vi "Test Parser Compatibility.vi"(8 "error in":errorcluster) -> (0 "error out":errorcluster)   [LabVIEW 2019]
uses:
  lvsrc/Classes/Parse/ParseVectorFile/ParseVectorFile.lvclass
  C:/Program Files (x86)/National Instruments/LabVIEW 2019/vi.lib/JKI/JKI SMO/SMO/SMO.lvclass
  <vilib>/addons/_JKI Toolkits/Caraya/classes/Assert/Assert True.vi
  <vilib>/Utility/AggHandler/Cls_AggHandler.xnode
  lvsrc/subVIs/typedefs/Parsed Path - Cluster.ctl
  <vilib>/Analysis/Matrix/Datatypes/RealMatrix.ctl
  lvsrc/subVIs/typedefs/Parsed Funnel - Cluster.ctl
  lvsrc/subVIs/typedefs/Parsed Rect - Cluster.ctl
  lvsrc/Classes/Parse/Dot/Dot.lvclass
  <vilib>/JKI/JKI SMO/SMO/SMO.lvclass
  <vilib>/addons/_JKI Toolkits/Caraya/classes/Test/Test.lvclass
  <vilib>/addons/_JKI Toolkits/Caraya/classes/Assert/Assert.lvclass
  <vilib>/Analysis/Matrix/NI_Matrix.lvlib
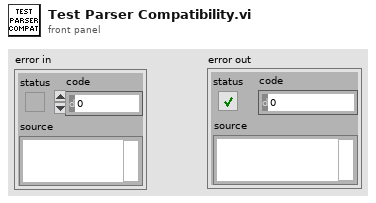
[diagram p1: front panel]
types:
  T1 = typedef "ParseVectorFile.lvclass/PublicEvents--ParseVectorFile.ParsedData.ctl" = cluster{"Paths":refnum<class "Path.lvclass">[], "Rectangles":refnum<class "Rectangle.lvclass">[], "SVGImage":refnum<class "SVGImage.lvclass">, "Dots":refnum<class "Dot.lvclass">[]}
  T2 = typedef "Parsed Path - Cluster.ctl" = cluster{"Fill Color":string, "Stroke Color":string, "Commands":cluster{"Command Type":string, "Coordinates":cluster{"X":dbl, "Y":dbl}[]}[], "Transformation Matrix":T3}
  T3 = typedef "NI_Matrix.lvlib/RealMatrix.ctl" = dbl[][]
  T4 = typedef "Parsed Funnel - Cluster.ctl" = cluster{"Fill Color":string, "Stroke Color":string, "Commands":cluster{"Command Type":string, "Coordinates":cluster{"X":dbl, "Y":dbl}[]}[], "Transformation Matrix":T3}
  T5 = typedef "Parsed Rect - Cluster.ctl" = cluster{"Fill":string, "Stroke":string, "width":dbl, "height":dbl, "x":dbl, "y":dbl, "Transformation Matrix":T3}
  T6 = cluster{" paths":T2[], " funnels":T4[], "rects":T5[], "Dots":refnum<class "Dot.lvclass">[]}
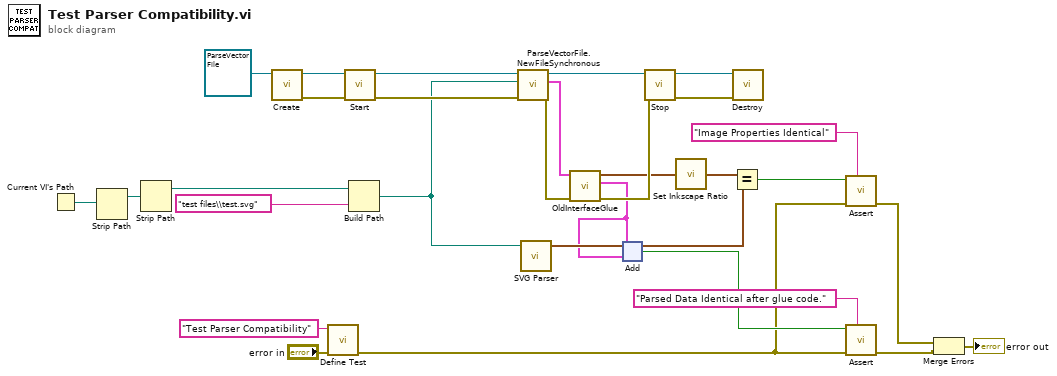
[diagram p0: block diagram]
diagram:
  n1 = Current VI's Path() -> (path=w17:path)
  n2 = Strip Path(path=w17) -> (stripped path=w16:path)  [unwired: 1 out]
  n3 = Strip Path(path=w16) -> (stripped path=w15:path)  [unwired: 1 out]
  n4 = call <vilib>:"Create.vi"("SMO"=refnum<class "ParseVectorFile.lvclass"> refnum ("ParseVectorFile.lvclass")) -> ("error out"=w28:errorcluster, "SMO out"=w29:refnum<class "ParseVectorFile.lvclass">)  [unwired: 8 in, 1 out]
  n5 = call <vilib>:"Define Test.vi"("error in (no error)"="error in", "Label (VI Title)"="Test Parser Compatibility") -> ("error out"=w6:errorcluster)  [unwired: 8 in, 1 out]
  n6 = call <vilib>:"Start.vi"("error in (no error)"=w28, "SMO"=w29) -> ("error out"=w19:errorcluster, "SMO out"=w25:refnum<class "ParseVectorFile.lvclass">)  [unwired: 8 in]
  n7 = Build Path(base path=w15, name or relative path="test files\\test.svg") -> (appended path=w13:path)
  n8 = call "ParseVectorFile.NewFileSynchronous.vi"("error in (no error)"=w19, "Path"=w13, "ParseVectorFile"=w25) -> ("error out"=w22:errorcluster, "ParsedData"=w23:T1, "ParseVectorFile out"=w24:refnum<class "ParseVectorFile.lvclass">)  [unwired: 6 in]
  n9 = call "SVG Parser.vi"("XML File Path"=w13) -> ("Image Size"=w2:cluster{"Width":dbl, "Height":dbl})  [unwired: 2 in, 2 out]
  n10 = call "OldInterfaceGlue.vi"("error in (no error)"=w22, "ParsedData"=w23) -> ("error out"=w21:errorcluster, "Parsing Data"=w1:T6, "Image Size"=w20:cluster{"Width":dbl, "Height":dbl})  [unwired: 7 in]
  n11 = xnode "Add"("Y"=w1, "X"=w1) -> ("Z"=w10:bool)
  n12 = call <vilib>:"Stop.vi"("error in (no error)"=w21, "SMO"=w24) -> ("error out"=w26:errorcluster, "SMO out"=w27:refnum<class "ParseVectorFile.lvclass">)  [unwired: 8 in]
  n13 = call "Set Inkscape Ratio.vi"("Image Size In"=w20) -> ("Image Size Out"=w18:cluster{"Width":dbl, "Height":dbl})
  n14 = Equal?(x=w18, y=w2) -> (x = y?=w12:bool)
  n15 = call <vilib>:"Destroy.vi"("error in (no error)"=w26, "SMO"=w27) -> ()  [unwired: 9 in, 1 out]
  n16 = call-poly <vilib>:"Assert.vi"("Label"="Image Properties Identical", "error in (no error)"=w6, "True?"=w12) -> ("error out"=w7:errorcluster)  [unwired: 7 in, 1 out]
  n17 = call-poly <vilib>:"Assert.vi"("Label"="Parsed Data Identical after glue code.", "error in (no error)"=w6, "True?"=w10) -> ("error out"=w8:errorcluster)  [unwired: 7 in, 1 out]
  n18 = Merge Errors(w7, w8) -> (→"error out":errorcluster)
